vi "Edit Cell.vi"(8 "error in (no error)":errorcluster, 10 "Display State In":T1, 11 "MCListbox Refnum":refnum<vi>) -> (0 "error out":errorcluster, 2 "Display State out":T1, 3 "MCListbox Refnum out":refnum<vi>)   [LabVIEW 2012, in "ListBox_XControl.xctl"]
doc: "Get MC Listbox Item names and column headers and put them into the X control properties.\nAlso turn ordering off."
uses:
  ListBox_XControl.xctl
  ListBox_State.ctl
  Order Type Def.ctl
  Value Filters.ctl
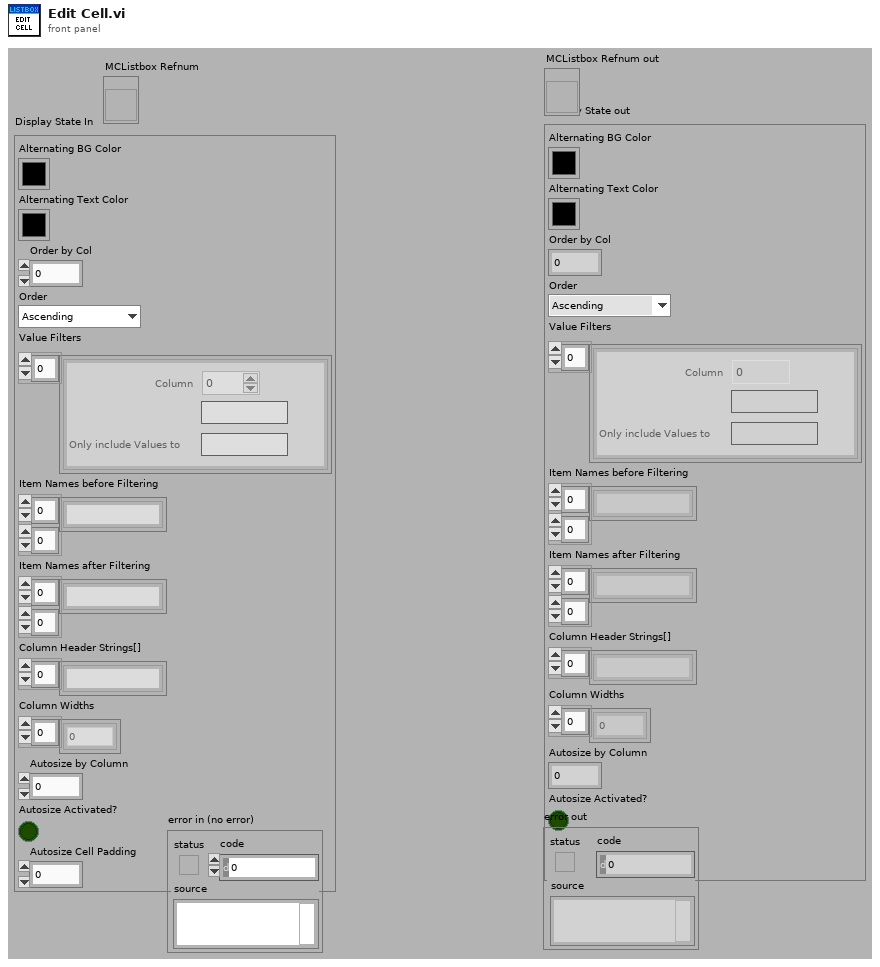
[diagram p1: front panel]
types:
  T1 = typedef "ListBox_XControl.xctl/ListBox_State.ctl" = cluster{"Alternating BG Color":u32, "Alternating Text Color":u32, "Order by Col":i32, "Order":T2, "Value Filters":T3, "Item Names before Filtering":string[][], "Item Names after Filtering":string[][], "Column Header Strings[]":string[], "Column Widths":u32[], "Autosize by Column":i32, "Autosize Activated?":bool, "Autosize Cell Padding":u32}
  T2 = typedef "ListBox_XControl.xctl/Order Type Def.ctl" = enum16{"Ascending", "Descending", "Off"}
  T3 = typedef "ListBox_XControl.xctl/Value Filters.ctl" = cluster{"Column":i32, "Only include Values From":string, "Only include Values to":string}[]
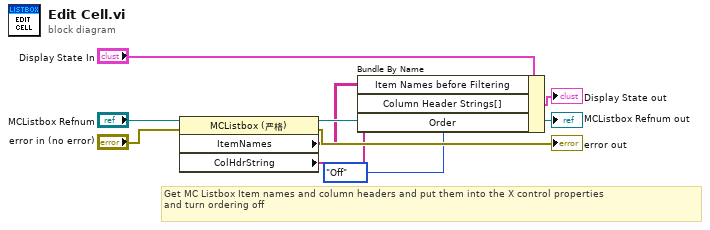
[diagram p0: block diagram]
diagram:
  # "Get MC Listbox Item names and column headers and put them into the X control properties\nand turn ordering off"
  n1 = property on="Property Node" class="MCListbox (严格)"(reference="MCListbox Refnum", error in="error in (no error)") -> (reference out=→"MCListbox Refnum out":refnum<vi>, error out=→"error out":errorcluster, "ItemNames"=w2:string[][], "ColHdrString"=w3:string[])
  n2 = Bundle By Name(cluster="Display State In", "Item Names before Filtering"=w2, "Column Header Strings[]"=w3, "Order"=Order_Type_Def."Off") -> (→"Display State out":T1)
